vi "hse-application_SetUserDefinedPath.vi"(8 "error in":errorcluster, 10 "Path":path, 11 "Name":string) -> (0 "error out":errorcluster)   [LabVIEW 2022 SP3, in "hse-application.lvclass"]
doc: "saves a user defined path with the specified name\n\n____\nHAMPEL SOFTWARE ENGINEERING v3.8.0 (2023-12-18 14:41)"
uses:
  hse-application.lvclass
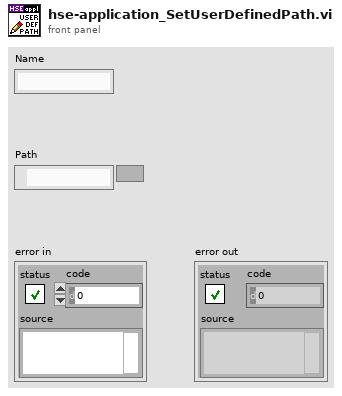
[diagram p1: front panel]
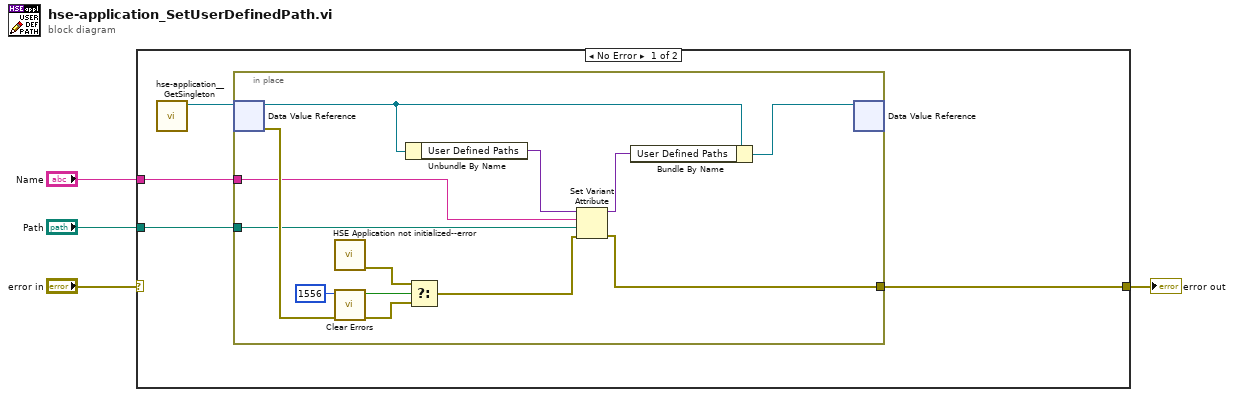
[diagram p0: block diagram]
diagram:
  n1 = case shown="No Error" "error in" {
    selector: "error in" -> [_ w22]
    tunnel: [w8 w22] -> w3
    tunnel: "Name" -> [w7 _]
    tunnel: "Path" -> [w6 _]
    frame No Error {
      n2 = call "hse-application__GetSingleton.vi"() -> ("ApplicationClass DVR"=w5:refnum<data-value>)  [unwired: 10 in, 1 out]
      n3 = in-place "In Place Element Structure" {
        in-place-border: [w21] -> w8
        in-place-border: w7 -> [w14]
        in-place-border: w6 -> [w13]
        n4 = in-place-dvr #1(w5) -> (w12:refnum<class "hse-application.lvclass">, w18:errorcluster)
        n5 = call "HSE Application not initialized--error.vi"() -> ("error out"=w20:errorcluster)  [unwired: 11 in]
        n6 = call <vilib>:"Clear Errors.vi"("error in (no error)"=w18, "specific error code to clear (0: all)"=1556) -> ("error out"=w19:errorcluster, "specific error cleared?"=w9:bool)  [unwired: 4 in]
        n7 = Unbundle By Name(w12) -> ("User Defined Paths"=w16:variant)
        n8 = Select(t=w20, s=w9, f=w19) -> (s? t:f=w17:errorcluster)
        n9 = Set Variant Attribute(Variant=w16, name=w14, value=w13, error in=w17) -> (Variant out=w15:variant, error out=w21:errorcluster)  [unwired: 1 out]
        n10 = Bundle By Name(cluster=w12, "User Defined Paths"=w15) -> (w11:refnum<class "hse-application.lvclass">)
        n11 = in-place-dvr #1(w11) -> ()  [unwired: 2 out]
      }
    }
    frame Error {
    }
  }
  "error out" <- w3
